vi "Destroy.vi"(11 "通知器输入":refnum<notifier>) -> (0 "错误输出":errorcluster)   [LabVIEW 2018, in "DataDisplay.lvlib"]
uses:
  DataDisplay.lvlib
  TypeDefine/DD_DataStream.ctl
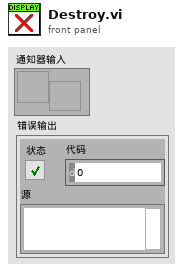
[diagram p1: front panel]
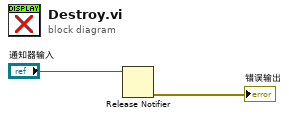
[diagram p0: block diagram]
diagram:
  n1 = Release Notifier(notifier="通知器输入") -> (error out=→"错误输出":errorcluster)  [unwired: 2 in, 2 out]
